vi "Read Memory.vi"(6 "Reverse Output[F]":bool, 8 "length (Byte, max. 16)":i32=16 max=16 step=1, 9 "offset (Byte, max. 16)":i32 max=16 step=1, 10 "Page Address":i32 format="%x", 11 "PN532 COM Port":refnum<visa-resource-name>) -> (0 "error out":errorcluster, 1 "Selected substring (HEX)":string, 2 "16-byte data(Hex)":string, 3 "PN532 COM Port Out":refnum<visa-resource-name>, 4 "Selected substring (ASCII)":string)   [LabVIEW 2012, in "NFC Driver.lvlib"]
doc: "This VI reads the 4 pages starting on the one specified by \"Address\"; i.e. If \"Address\" is 0x00 then \"16-byte data\" will return the data in pages 0x00, 0x01, 0x02 and 0x03.\n\nIt is possible to specify to get a subset of the information stored in the returned pages by using \"offset (max. 16) and \"length (max. 16)\". The desired subset of information will be returned in \"Selected substring (HEX)\" (raw hex format) and \"Selected substring (ASCII)\" (ASCII format)."
uses:
  NFC Driver.lvlib
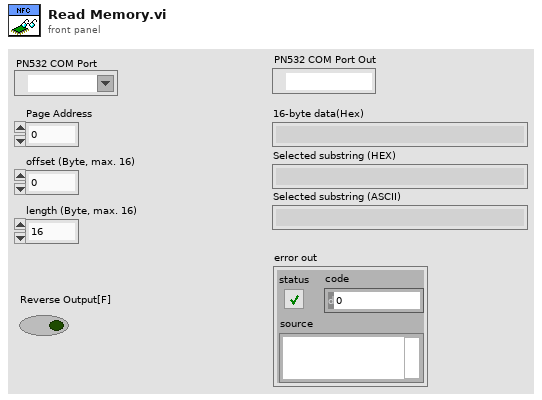
[diagram p1: front panel]
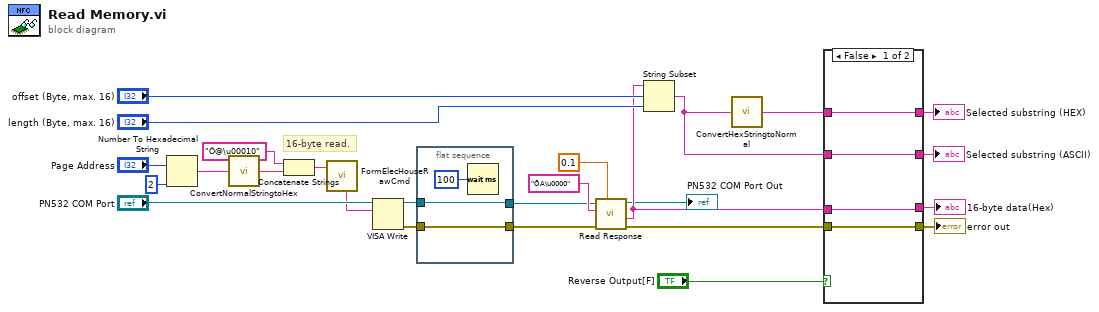
[diagram p0: block diagram]
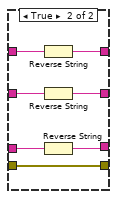
[diagram p2: hidden frame]
diagram:
  # "16-byte read."
  n1 = Number To Hexadecimal String(1:i16 2 ("width (-)"), 2:"Page Address") -> (0:w12:string)
  n2 = call "ConvertNormalStringtoHex.vi"("Normal String"=w12) -> ("Hex String"=w14:string)
  n3 = Concatenate Strings("Ô@\u00010" ("string"), w14) -> (w25:string)
  n4 = call "FormElecHouseRawCmd.vi"("Command"=w25) -> ("concatenated Cmd"=w23:string)  [unwired: 10 in]
  n5 = VISA Write(VISA resource name="PN532 COM Port", write buffer=w23) -> (VISA resource name out=w18:refnum<visa-resource-name>, error out=w16:errorcluster)  [unwired: 1 in, 1 out]
  n6 = flat-sequence {
    tunnel: w18 -> [w28]
    tunnel: [w28] -> w17
    tunnel: w16 -> [w27]
    tunnel: [w27] -> w15
    frame #0 {
      n7 = Wait (ms)(milliseconds to wait=u32 100) -> ()  [unwired: 1 out]
    }
  }
  n8 = call "Read Response.vi"("Timeout (s)"=0.1, "error in (no error)"=w15, "regular expression"="ÕA\u0000", "PN532 COM Port"=w17) -> ("error out"=w6:errorcluster, "Response Data"=w8:string, "PN532 COM Port Out"=→"PN532 COM Port Out":refnum<visa-resource-name>)  [unwired: 4 in, 1 out]
  n9 = String Subset(string=w8, offset (0)="offset (Byte, max. 16)", length (rest)="length (Byte, max. 16)") -> (substring=w4:string)
  n10 = call "ConvertHexStringtoNormal.vi"("Hex String"=w4) -> ("Normal String"=w3:string)
  n11 = case shown="False" "Reverse Output[F]" {
    tunnel: [w33 w37] -> w11
    tunnel: w3 -> [w33 w40]
    tunnel: [w32 w36] -> w10
    tunnel: w4 -> [w32 w39]
    tunnel: [w31 w35] -> w7
    tunnel: w8 -> [w31 w38]
    tunnel: w6 -> [w30 w34]
    tunnel: [w30 w34] -> w5
    frame False {
    }
    frame True {
      n12 = Reverse String(1:w40) -> (0:w37:string)
      n13 = Reverse String(1:w39) -> (0:w36:string)
      n14 = Reverse String(1:w38) -> (0:w35:string)
    }
  }
  "error out" <- w5
  "16-byte data(Hex)" <- w7
  "Selected substring (HEX)" <- w11
  "Selected substring (ASCII)" <- w10
